vi "Test CTIWrapper API.vi"() -> ()   [LabVIEW 2024]
doc: "CTIWrapper API Tester."
uses:
  <instrlib>/HandsOnPi2040/cti-drivers-lv-visa-main/CTI-Visa/Identity.ctl
  <vilib>/Utility/error.llb/DialogType.ctl
  CTIWrapper.lvlib
  <instrlib>/HandsOnPi2040/cti-drivers-lv-visa-main/CTI-Visa/CTI-Visa.lvlib
panel:
  in  "Close Device":bool
  out "Digital Inputs":map{i32, bool[]}(c390)
  in  "Digital Outputs":bool[](array[boolean])
  in  "Set DO":bool
  out "Connection Status":bool
  out "Identity":T1
  in  "VISA resource name":refnum<visa-resource-name>
  in  "Initialize Device":bool
  out "last error":errorcluster
  in  "Show Diagram on Init":bool
  in  "Run as Singleton?":bool
  in  "Show Block Diagram":bool
  in  "Refresh Modules":bool
  out "Active Modules":string[](array[string])
  in  "Stop Module":bool
  in  "Select Module":i32(ring)=-1 caption="Select Module\nTo send Request to" items=["All"=-1]
  in  "Run New Module":bool
  in  "Hide Module Panel":bool
  in  "Show Module Panel":bool
  out "Status":string
  # "This VI tests the API for the Module."
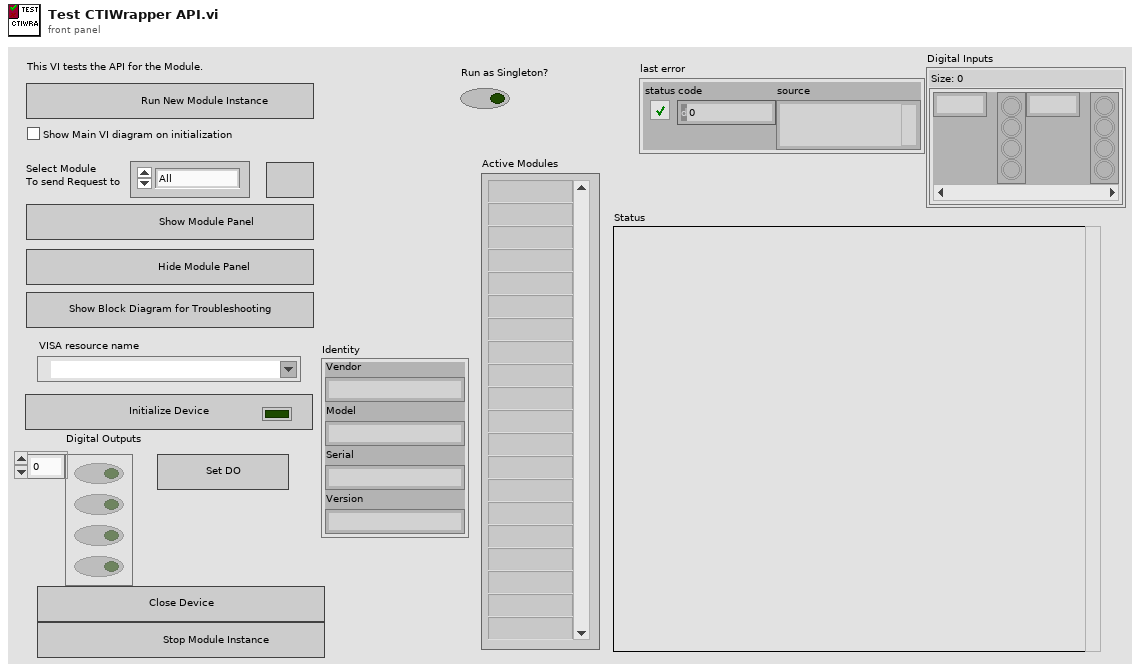
[diagram p1: front panel]
types:
  T1 = typedef "CTI-Visa.lvlib/Identity.ctl" = cluster{"Vendor":string, "Model":string, "Serial":string, "Version":string}
  T2 = typedef "CTIWrapper.lvlib/Broadcast Events--cluster.ctl" = cluster{"Module Did Init":refnum<user-event>, "Status Updated":refnum<user-event>, "Error Reported":refnum<user-event>, "Module Did Stop":refnum<user-event>, "Update Module Execution Status":refnum<user-event>, "Connection Status Updated":refnum<user-event>, "Digital Inptus Updated":refnum<user-event>}
  T3 = typedef "DialogType.ctl" = u16
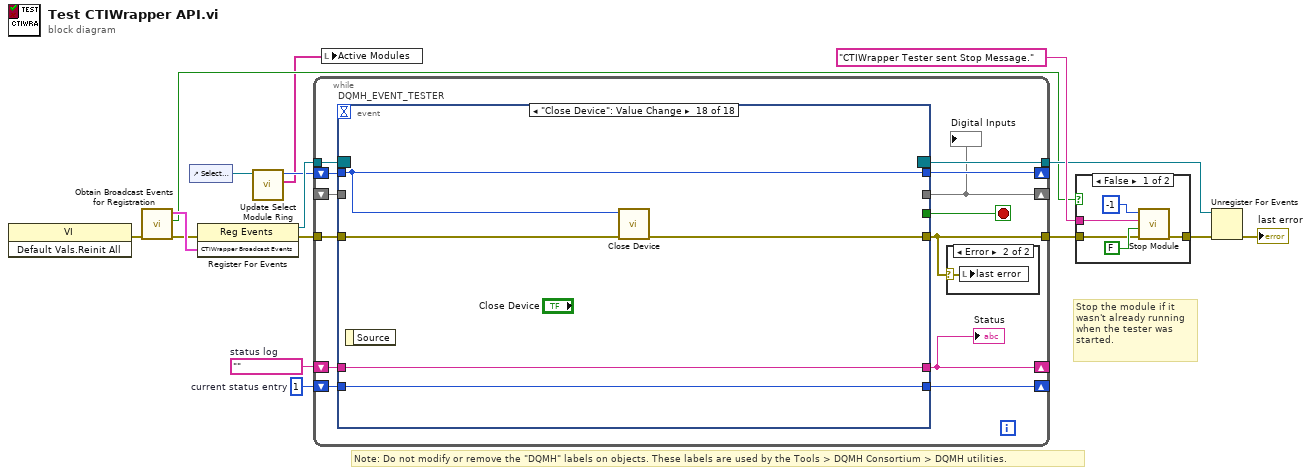
[diagram p0: block diagram]
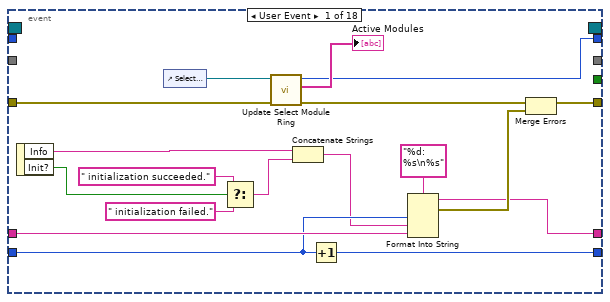
[diagram p4: hidden frame]
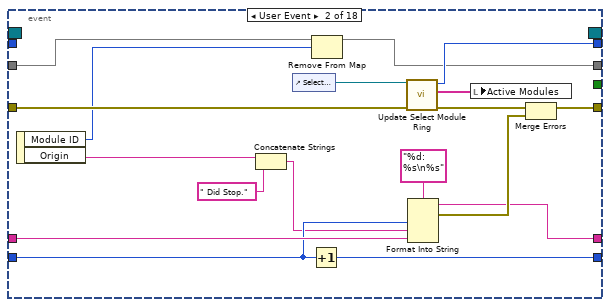
[diagram p5: hidden frame]
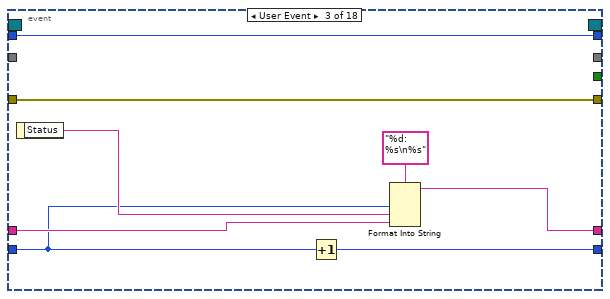
[diagram p6: hidden frame]
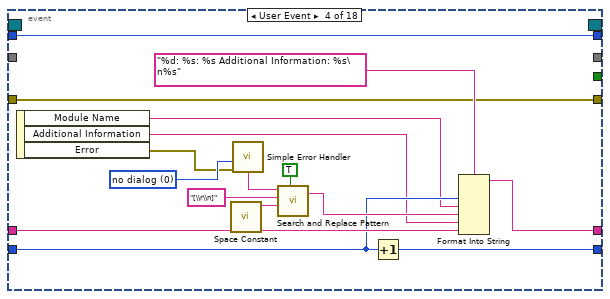
[diagram p7: hidden frame]
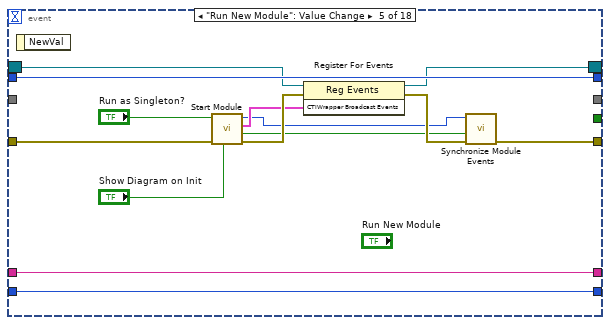
[diagram p8: hidden frame]
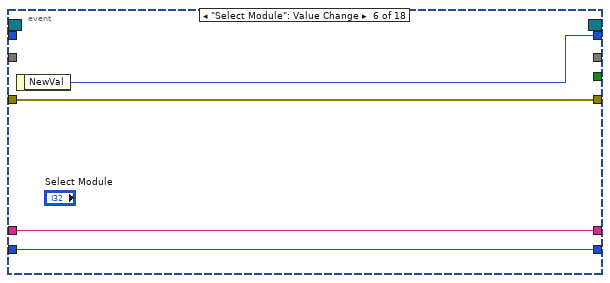
[diagram p9: hidden frame]
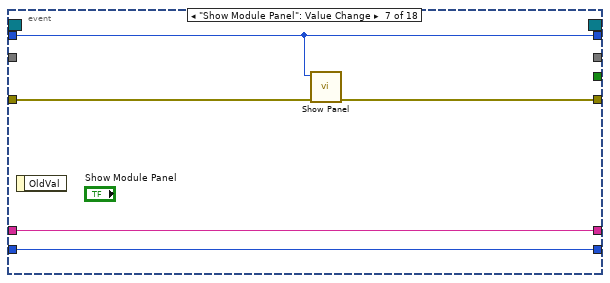
[diagram p10: hidden frame]
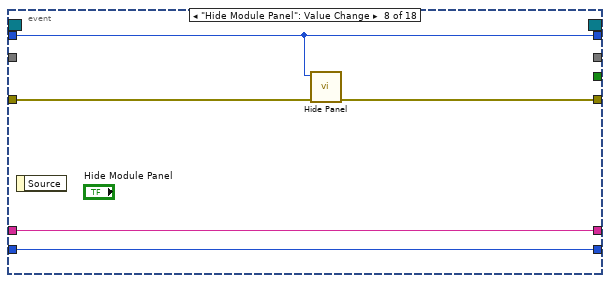
[diagram p11: hidden frame]
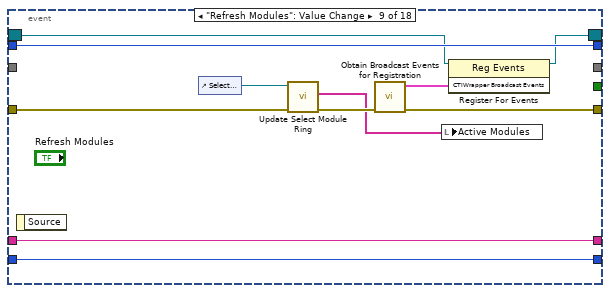
[diagram p12: hidden frame]
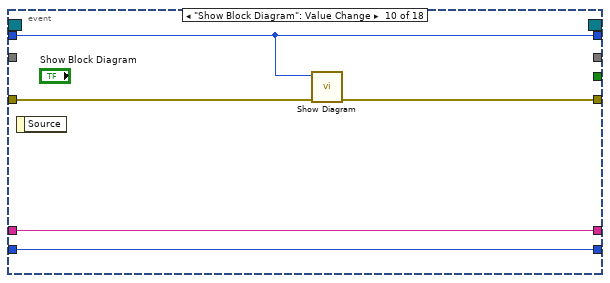
[diagram p13: hidden frame]
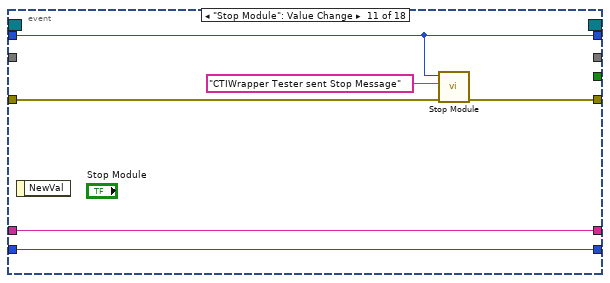
[diagram p14: hidden frame]
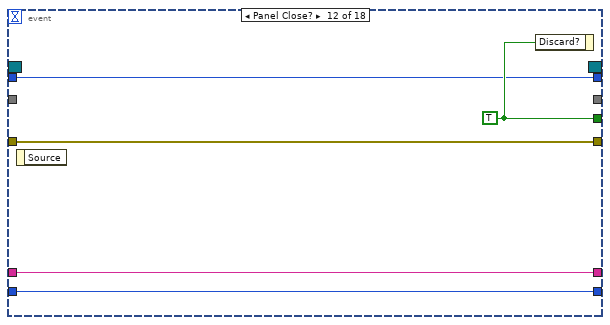
[diagram p15: hidden frame]
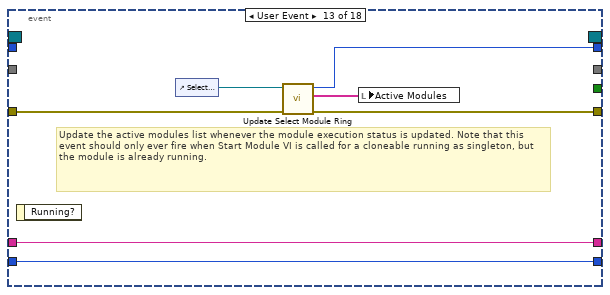
[diagram p16: hidden frame]
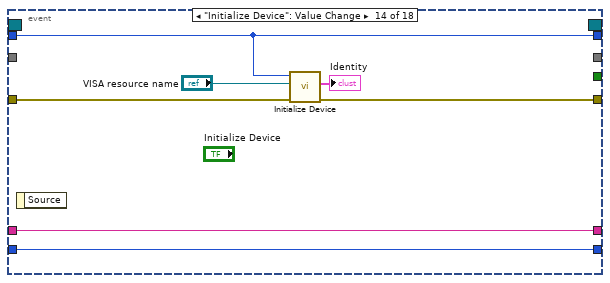
[diagram p17: hidden frame]
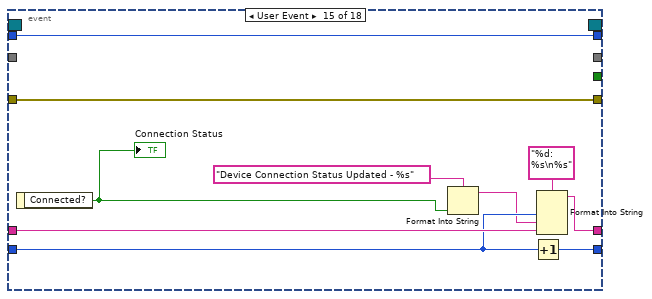
[diagram p18: hidden frame]
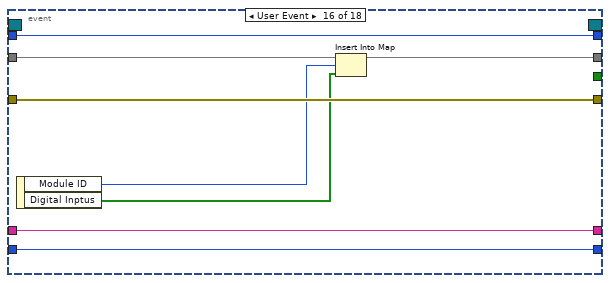
[diagram p19: hidden frame]
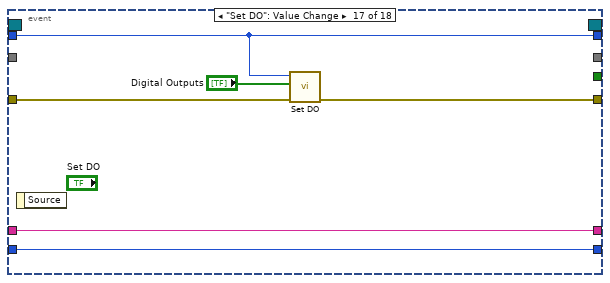
[diagram p20: hidden frame]
diagram:
  w13 = 1  # current status entry
  w14 = ""  # status log
  # "Stop the module if it wasn't already running when the tester was started."
  # "Note: Do not modify or remove the \"DQMH\" labels on objects. These labels are used by the Tools > DQMH Consortium > DQMH utilities."
  n1 = invoke class="VI" method="Default Vals.Reinit All"() -> (error out=w8:errorcluster)  [unwired: 3 in, 2 out]
  n2 = call "Obtain Broadcast Events for Registration.vi"("error in"=w8) -> ("error out"=w7:errorcluster, "Already running?"=w6:bool, "CTIWrapper Broadcast Events"=w12:T2)  [unwired: 8 in]
  n3 = control-ref of="Select Module"() -> (w3:refnum<vi>)
  n4 = register-events(error in=w7, w12) -> (reference out=w16:refnum<event-registration>, error out=w11:errorcluster)  [unwired: 1 in]
  n5 = call "Update Select Module Ring.vi"("Select Module Ring Ref"=w3) -> ("Active Modules (Array)"=w1:string[], "New Module Ring Value"=w2:i32)  [unwired: 8 in, 1 out]
  n6 = while {
    tunnel: w16 -> [w29]
    tunnel: [w20] -> w5
    tunnel: w11 -> [w28]
    shift-right: [w24] -> _
    shift-left: w14 -> [w26]
    shift-right: [w25] -> _
    shift-left: w13 -> [w27]
    shift-right: [w22] -> _
    shift-left: w2 -> [w23]
    tunnel: [w21] -> w9
    shift-right: [w18] -> _
    shift-left: _ -> [w17]
    stop <- w19 stop-if-true
    n7 = event "DQMH_EVENT_TESTER" shown="[17] \"Close Device\": Value Change" {
      selector: w29 -> [_ _ _ _ w98 _ _ _ w124 _ _ _ _ _ _ _ _ _]
      dyn-events: [_ _ _ _ w97 _ _ _ w123 _ _ _ _ _ _ _ _ _] -> w21
      timeout: _ -> [_ _ _ _ _ _ _ _ _ _ _ _ _ _ _ _ _ _]
      tunnel: [_ _ _ _ _ _ _ _ _ _ _ w145 _ _ _ _ _ _] -> w19
      tunnel: [w38 w58 w74 w78 w96 w108 w112 w117 w120 w131 w136 w144 w148 w155 w169 w177 w179 w184] -> w20
      tunnel: w28 -> [w40 w60 w74 w78 w99 w108 w113 w118 w125 w134 w137 w144 w149 w159 w169 w177 w183 w188]
      tunnel: w27 -> [w45 w63 w67 w81 w101 w106 w110 w115 w128 w132 w139 w142 w151 w157 w165 w174 w181 w186]
      tunnel: w26 -> [w46 w64 w70 w82 w102 w107 w111 w116 w129 w133 w140 w143 w152 w158 w167 w175 w182 w187]
      tunnel: [w43 w61 w71 w80 w102 w107 w111 w116 w129 w133 w140 w143 w152 w158 w166 w175 w182 w187] -> w24
      tunnel: [w44 w62 w73 w79 w101 w106 w110 w115 w128 w132 w139 w142 w151 w157 w164 w174 w181 w186] -> w25
      tunnel: w23 -> [_ _ w68 w90 w100 _ w109 w114 w127 w130 w138 w141 _ w156 w168 w176 w180 w185]
      tunnel: [w35 w55 w68 w90 w100 w105 w109 w114 w127 w130 w138 w141 w147 w156 w168 w176 w180 w185] -> w22
      tunnel: [_ w50 _ _ _ _ _ _ _ _ _ _ _ _ _ w171 _ _] -> w18
      tunnel: w17 -> [_ w51 _ _ _ _ _ _ _ _ _ _ _ _ _ w170 _ _]
      event User Event {
        n8 = event-data() -> ("Info"=w42:string, "Init?"=w32:bool)  [unwired: 1 in]
        n9 = control-ref of="Select Module"() -> (w37:refnum<vi>)
        n10 = Select(t=" initialization succeeded.", s=w32, f=" initialization failed.") -> (s? t:f=w31:string)
        n11 = call "Update Select Module Ring.vi"("error in"=w40, "Select Module Ring Ref"=w37) -> ("error out"=w39:errorcluster, "Active Modules (Array)"=→"Active Modules":string[], "New Module Ring Value"=w35:i32)  [unwired: 7 in]
        n12 = Concatenate Strings(w42, w31) -> (w41:string)
        n13 = Increment(x=w45) -> (x+1=w44:i32)
        n14 = Format Into String(format string="%d: %s\n%s", w45, w41, w46) -> (resulting string=w43:string, error out=w48:errorcluster)  [unwired: 2 in]
        n15 = Merge Errors(w39, w48) -> (w38:errorcluster)
      }
      event User Event {
        n16 = event-data() -> ("Module ID"=w49:i32, "Origin"=w53:string)  [unwired: 1 in]
        n17 = Concatenate Strings(w53, " Did Stop.") -> (w52:string)
        n18 = control-ref of="Select Module"() -> (w57:refnum<vi>)
        n19 = Increment(x=w63) -> (x+1=w62:i32)
        n20 = Remove From Map(10:w49, 11:w51) -> (3:w50:map{i32, bool[]})  [unwired: 2 out]
        n21 = call "Update Select Module Ring.vi"("error in"=w60, "Select Module Ring Ref"=w57) -> ("error out"=w59:errorcluster, "Active Modules (Array)"=w56:string[], "New Module Ring Value"=w55:i32)  [unwired: 7 in]
        n22 = Format Into String(format string="%d: %s\n%s", w63, w52, w64) -> (resulting string=w61:string, error out=w66:errorcluster)  [unwired: 2 in]
        n23 = local write "Active Modules"(w56) -> ()
        n24 = Merge Errors(w59, w66) -> (w58:errorcluster)
      }
      event User Event {
        n25 = event-data() -> ("Status"=w69:string)  [unwired: 1 in]
        n26 = Increment(x=w67) -> (x+1=w73:i32)
        n27 = Format Into String(format string="%d: %s\n%s", w67, w69, w70) -> (resulting string=w71:string)  [unwired: 2 in, 1 out]
      }
      event User Event {
        w83 = T3 0 items=["no dialog", "OK message", "continue or stop message", "OK message + warnings", "continue/stop + warnings"] ("type of dialog (OK msg:1)")
        n28 = event-data() -> ("Module Name"=w77:string, "Additional Information"=w76:string, "Error"=w75:errorcluster)  [unwired: 1 in]
        n29 = call <vilib>:"Space Constant.vi"() -> ("String"=w87:string)
        n30 = call <vilib>:"Simple Error Handler.vi"("type of dialog (OK msg:1)"=w83, "error in (no error)"=w75) -> ("message"=w84:string)  [unwired: 3 in, 4 out]
        n31 = call <vilib>:"Search and Replace Pattern.vi"("string"=w84, "regular expression (\"\")"="[\\r\\n]" ("regular expression (\"\")"), "replace string (\"\")"=w87, "replace all? (F)"=TRUE ("replace all CR/LF with spaces")) -> ("result string"=w85:string)  [unwired: 1 in, 1 out]
        n32 = Increment(x=w81) -> (x+1=w79:i32)
        n33 = Format Into String(format string="%d: %s: %s Additional Information: %s\n%s", w81, w77, w85, w76, w82) -> (resulting string=w80:string)  [unwired: 2 in, 1 out]
      }
      event "Run New Module": Value Change {
        n34 = event-data() -> ()  [unwired: 1 in, 1 out]
        n35 = call "Start Module.vi"("Show Main VI Diagram on Init (F)"="Show Diagram on Init", "error in"=w99, "Run as Singleton? (F)"="Run as Singleton?") -> ("error out"=w103:errorcluster, "Wait for Event Sync?"=w95:bool, "CTIWrapper Broadcast Events"=w94:T2, "Module ID"=w91:i32)  [unwired: 4 in, 1 out]
        n36 = register-events(reference=w98, error in=w103, w94) -> (reference out=w97:refnum<event-registration>, error out=w104:errorcluster)
        n37 = call "Synchronize Module Events.vi"("error in"=w104, "Wait for Event Sync?"=w95, "Module ID in"=w91) -> ("error out"=w96:errorcluster)  [unwired: 7 in, 1 out]
      }
      event "Select Module": Value Change {
        n38 = event-data() -> ("NewVal"=w105:i32)  [unwired: 1 in]
      }
      event "Show Module Panel": Value Change {
        n39 = event-data() -> ()  [unwired: 1 in, 1 out]
        n40 = call "Show Panel.vi"("error in"=w113, "Module ID"=w109) -> ("error out"=w112:errorcluster)  [unwired: 9 in]
      }
      event "Hide Module Panel": Value Change {
        n41 = event-data() -> ()  [unwired: 1 in, 1 out]
        n42 = call "Hide Panel.vi"("error in"=w118, "Module ID"=w114) -> ("error out"=w117:errorcluster)  [unwired: 9 in]
      }
      event "Refresh Modules": Value Change {
        n43 = event-data() -> ()  [unwired: 1 in, 1 out]
        n44 = control-ref of="Select Module"() -> (w126:refnum<vi>)
        n45 = call "Update Select Module Ring.vi"("error in"=w125, "Select Module Ring Ref"=w126) -> ("error out"=w121:errorcluster, "Active Modules (Array)"=w119:string[])  [unwired: 7 in, 1 out]
        n46 = call "Obtain Broadcast Events for Registration.vi"("error in"=w121) -> ("error out"=w120:errorcluster, "CTIWrapper Broadcast Events"=w122:T2)  [unwired: 8 in, 1 out]
        n47 = local write "Active Modules"(w119) -> ()
        n48 = register-events(reference=w124, w122) -> (reference out=w123:refnum<event-registration>)  [unwired: 1 in, 1 out]
      }
      event "Show Block Diagram": Value Change {
        n49 = event-data() -> ()  [unwired: 1 in, 1 out]
        n50 = call "Show Diagram.vi"("error in"=w134, "Module ID"=w130) -> ("error out"=w131:errorcluster)  [unwired: 9 in]
      }
      event "Stop Module": Value Change {
        n51 = event-data() -> ()  [unwired: 1 in, 1 out]
        n52 = call "Stop Module.vi"("error in"=w137, "Origin"="CTIWrapper Tester sent Stop Message", "Module ID"=w138) -> ("error out"=w136:errorcluster)  [unwired: 8 in]
      }
      event Panel Close? {
        w145 = TRUE ("Discard?")
        n53 = event-data() -> ()  [unwired: 1 in, 1 out]
        n54 = event-data("Discard?"=w145) -> ()  [unwired: 1 in, 1 out]
      }
      event User Event {
        # "Update the active modules list whenever the module execution status is updated. Note that this event should only ever fire when Start Module VI is called for a cloneable running as singleton, but the module is already running."
        n55 = event-data() -> ()  [unwired: 1 in, 1 out]
        n56 = control-ref of="Select Module"() -> (w150:refnum<vi>)
        n57 = call "Update Select Module Ring.vi"("error in"=w149, "Select Module Ring Ref"=w150) -> ("error out"=w148:errorcluster, "Active Modules (Array)"=w146:string[], "New Module Ring Value"=w147:i32)  [unwired: 7 in]
        n58 = local write "Active Modules"(w146) -> ()
      }
      event "Initialize Device": Value Change {
        n59 = event-data() -> ()  [unwired: 1 in, 1 out]
        n60 = call "Initialize Device.vi"("error in"=w159, "VISA resource name"="VISA resource name", "Module ID"=w156) -> ("error out"=w155:errorcluster, "Identity"=→"Identity":T1)  [unwired: 6 in, 1 out]
      }
      event User Event {
        n61 = event-data() -> ("Connected?"=w160:bool)  [unwired: 1 in]
        "Connection Status" <- w160
        n62 = Format Into String(format string="Device Connection Status Updated - %s", w160) -> (resulting string=w161:string)  [unwired: 2 in, 1 out]
        n63 = Increment(x=w165) -> (x+1=w164:i32)
        n64 = Format Into String(format string="%d: %s\n%s", w165, w161, w167) -> (resulting string=w166:string)  [unwired: 2 in, 1 out]
      }
      event User Event {
        n65 = event-data() -> ("Module ID"=w173:i32, "Digital Inptus"=w172:bool[])  [unwired: 1 in]
        n66 = Insert Into Map(map in=w170, key=w173, value=w172) -> (map out=w171:map{i32, bool[]})  [unwired: 2 out]
      }
      event "Set DO": Value Change {
        n67 = event-data() -> ()  [unwired: 1 in, 1 out]
        n68 = call "Set DO.vi"("error in"=w183, "Digital Outputs"="Digital Outputs", "Module ID"=w180) -> ("error out"=w179:errorcluster)  [unwired: 8 in]
      }
      event "Close Device": Value Change {
        n69 = event-data() -> ()  [unwired: 1 in, 1 out]
        n70 = call "Close Device.vi"("error in"=w188, "Module ID"=w185) -> ("error out"=w184:errorcluster)  [unwired: 9 in]
      }
    }
    "Status" <- w24
    "Digital Inputs" <- w18
    n71 = case shown="Error" w20 {
      selector: w20 -> [_ w30]
      frame No Error {
      }
      frame Error {
        n72 = local write "last error"(w30) -> ()
      }
    }
  }
  n73 = local write "Active Modules"(w1) -> ()
  n74 = case shown="False" w6 {
    tunnel: [w193 w194] -> w15
    tunnel: "CTIWrapper Tester sent Stop Message." ("Origin") -> [w192 _]
    tunnel: w5 -> [w189 w194]
    frame False {
      n75 = call "Stop Module.vi"("error in"=w189, "Wait for Module to stop? (F)"=FALSE ("Wait for Module to stop?"), "Origin"=w192, "Module ID"=-1 ("Stop all")) -> ("error out"=w193:errorcluster)  [unwired: 7 in]
    }
    frame True {
    }
  }
  n76 = Unregister For Events(event registration refnum=w9, error in=w15) -> (error out=→"last error":errorcluster)
